vi "Barcode_decode.vi"(1 "Barcode data":u8[][](array[numeric]) format="%.0x") -> (0 "String 2":string)   [LabVIEW 2024, in "PCANusb_DTU.lvlib"]
uses:
  PCANusb_DTU.lvlib
panel:
  out "Array":string[](array[string])
  out "String":string
  out "array w/ subset deleted":u8[][](array[numeric]) format="%.0x"
  # "ADDGSC000001"
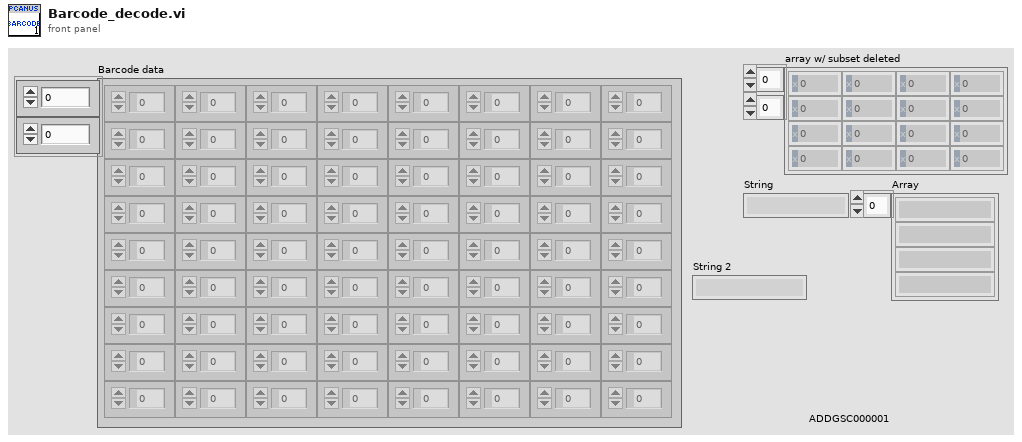
[diagram p1: front panel]
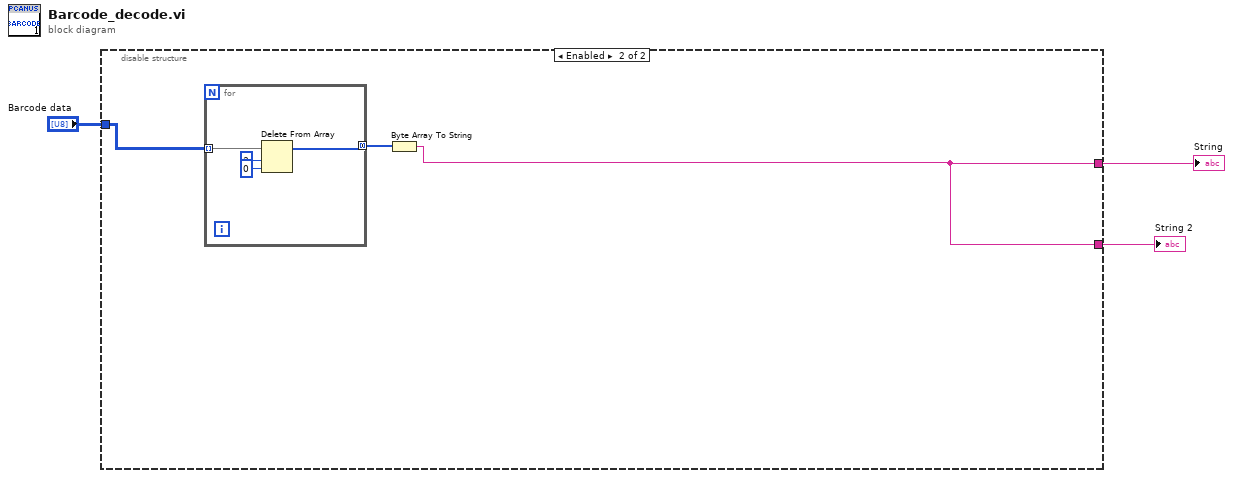
[diagram p0: block diagram]
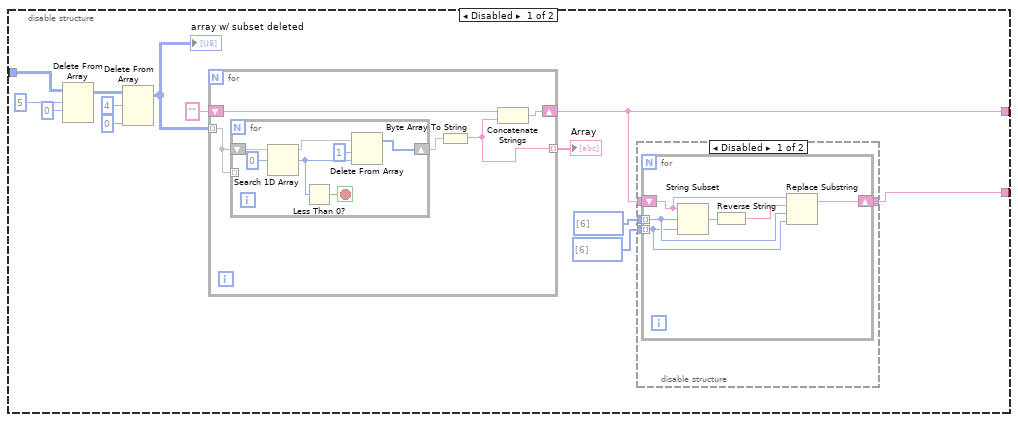
[diagram p2: hidden frame]
diagram:
  n1 = disable-structure shown="Enabled" {
    disable-tunnel: "Barcode data" -> [w16 w41]
    disable-tunnel: [w7 w39] -> w2
    disable-tunnel: [w4 w39] -> w1
    frame Disabled {
      n2 = Delete From Array(array=w16, length=5, index (row)=0) -> (array with subset deleted=w13:u8[][])  [unwired: 1 in, 1 out]
      n3 = Delete From Array(array=w13, length=4, index (col)=0 ("disabled index (col)")) -> (array with subset deleted=w10:u8[][])  [unwired: 1 in, 1 out]
      "array w/ subset deleted" <- w10
      n4 = for {
        tunnel: w10 -> [w29] mode=indexing
        shift-right: [w31] -> w7
        shift-left: "" -> [w32]
        tunnel: [w30] -> w8 mode=indexing
        n5 = for {
          tunnel: w29 -> [_] mode=indexing
          shift-right: [w35] -> w28
          shift-left: w29 -> [w36]
          stop <- w38 stop-if-true
          n6 = Search 1D Array(1D array=w36, element=u8 0) -> (index of element=w37:i32)  [unwired: 1 in]
          n7 = Less Than 0?(x=w37) -> (x < 0?=w38:bool)
          n8 = Delete From Array(array=w36, length=1, index=w37) -> (array with subset deleted=w35:u8[])  [unwired: 1 out]
        }
        n9 = Byte Array To String(unsigned byte array=w28) -> (string=w30:string)
        n10 = Concatenate Strings(w32, w30) -> (w31:string)
      }
      "Array" <- w8
      n11 = disable-structure shown="Disabled" {
        disable-tunnel: w7 -> [w20 w27]
        disable-tunnel: i32[] [6] ("length (rest)") -> [w19 _]
        disable-tunnel: i32[] [6] ("length (rest)") -> [w18 _]
        disable-tunnel: [w17 w27] -> w4
        frame Disabled {
          n12 = for {
            tunnel: w19 -> [w21] mode=indexing
            tunnel: w18 -> [w22] mode=indexing
            shift-right: [w25] -> w17
            shift-left: w20 -> [w24]
            n13 = String Subset(string=w24, offset (0)=w22, length (rest)=w21) -> (substring=w26:string)
            n14 = Reverse String(1:w26) -> (0:w23:string)
            n15 = Replace Substring(2:w21, 3:w22, 4:w23, 5:w24) -> (1:w25:string)  [unwired: 1 out]
          }
        }
        frame Enabled {
        }
      }
    }
    frame Enabled {
      n16 = for {
        tunnel: w41 -> [w45] mode=indexing
        tunnel: [w42] -> w40 mode=concatenating
        n17 = Delete From Array(array=w45, length=3, index=0) -> (array with subset deleted=w42:u8[])  [unwired: 1 out]
      }
      n18 = Byte Array To String(unsigned byte array=w40) -> (string=w39:string)
    }
  }
  "String" <- w2
  "String 2" <- w1
